vi "Generate Project Path from OS.vi"(10 "Plugin OS":T1, 11 "Project Path in":path) -> (3 "Project Path out":path)   [LabVIEW 2023, in "Plugin Generator.lvlib" / "PluginGenerator_MetaDataObj.lvclass"]
uses:
  PluginGenerator_MetaDataObj.lvclass
  Typedef/Plugin OS.ctl
  Plugin Generator.lvlib
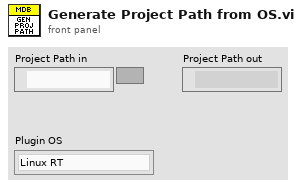
[diagram p1: front panel]
types:
  T1 = typedef "Plugin Generator.lvlib/Plugin OS.ctl" = enum16{"Linux RT", "Env Server"}
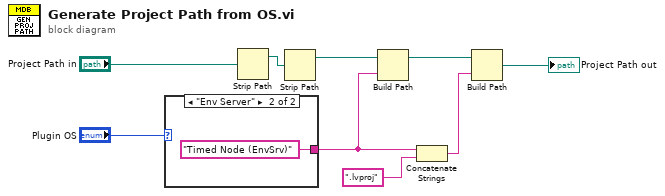
[diagram p0: block diagram]
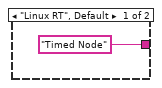
[diagram p2: hidden frame]
diagram:
  n1 = case shown="\"Env Server\"" "Plugin OS" {
    tunnel: ["Timed Node" "Timed Node (EnvSrv)"] -> w5
    frame "Linux RT", Default {
    }
    frame "Env Server" {
    }
  }
  n2 = Strip Path(path="Project Path in") -> (stripped path=w3:path)  [unwired: 1 out]
  n3 = Strip Path(path=w3) -> (stripped path=w4:path)  [unwired: 1 out]
  n4 = Build Path(base path=w4, name or relative path=w5) -> (appended path=w7:path)
  n5 = Concatenate Strings(w5, ".lvproj" ("string")) -> (w9:string)
  n6 = Build Path(base path=w7, name or relative path=w9) -> (appended path=→"Project Path out":path)
